vi "gracefulShutDown.vi"   [LabVIEW 2015]
uses:
  <vilib>/DAQmx/write.llb/DAQmx Write (Digital Bool 1Line 1Point).vi
  <vilib>/DAQmx/miscellaneous.llb/DAQmx Fill In Error Info.vi
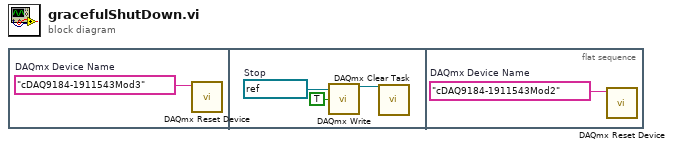
[diagram p0: block diagram]
diagram:
  n1 = flat-sequence {
    frame #0 {
      w1 = tag "cDAQ9184-1911543Mod3"  # DAQmx Device Name
      n2 = call <vilib>:"DAQmx Reset Device.vi"("device in"=w1) -> ()  [unwired: 14 in, 1 out]
    }
    frame #1 {
      w2 = refnum<k21> "DO1P1"  # Stop
      n3 = call-poly <vilib>:"DAQmx Write.vi"("task/channels in"=w2, "data"=TRUE) -> ("task out"=w3:refnum<k21>)  [unwired: 11 in, 2 out]
      n4 = call <vilib>:"DAQmx Clear Task.vi"("task in"=w3) -> ()  [unwired: 14 in, 1 out]
    }
    frame #2 {
      w5 = tag "cDAQ9184-1911543Mod2"  # DAQmx Device Name
      n5 = call <vilib>:"DAQmx Reset Device.vi"("device in"=w5) -> ()  [unwired: 14 in, 1 out]
    }
  }
